vi "Dripline-agent.vi"() -> ()   [LabVIEW 2016]
panel:
  in  "message":string
  in  "target":string
  in  "timeout":dbl=10.0 format="%#_13g"
  in  "value":string
  in  "endpoint":string="broadcast.ping"
  in  "Request op":u16(ring)=1 items=["Set"=0, "Get"=1, "Send"=7, "Run"=8, "Command"=9]
  in  "Message type":u16(ring)=1 items=["alert", "request"]
  in  "host name":string="higgsino.physics.ucsb.edu"
  out "Array - String":string[](array[string])
  in  "error (in)":errorcluster
  out "error out":errorcluster
  # "alerts fields"
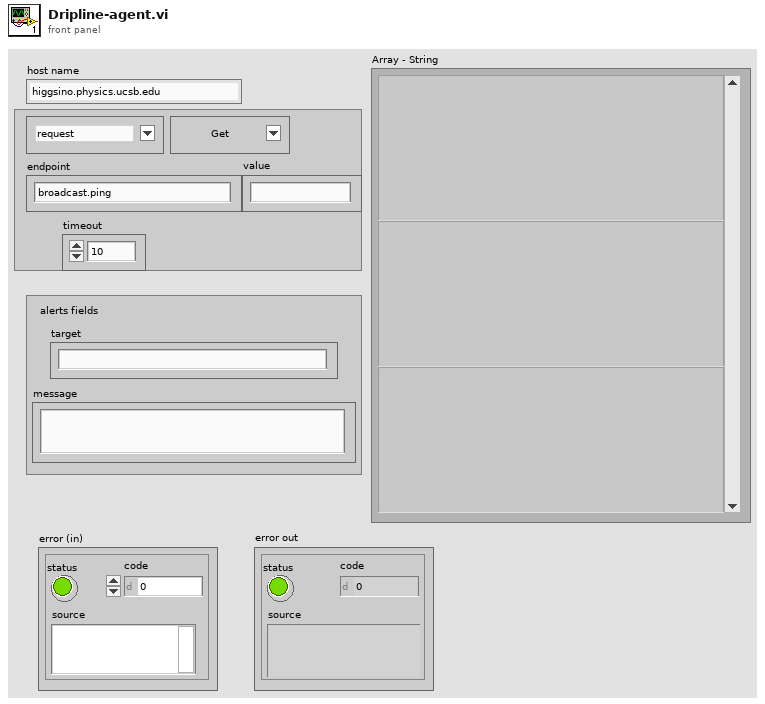
[diagram p1: front panel]
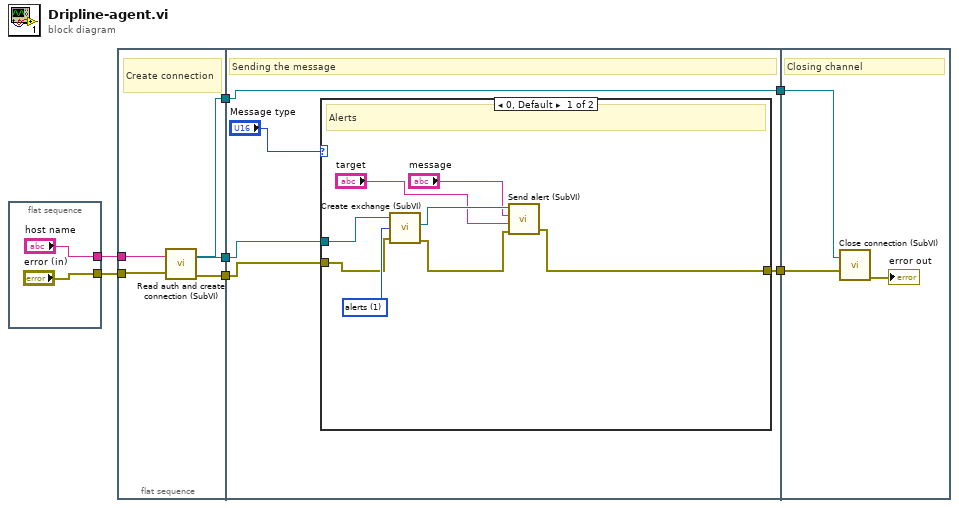
[diagram p0: block diagram]
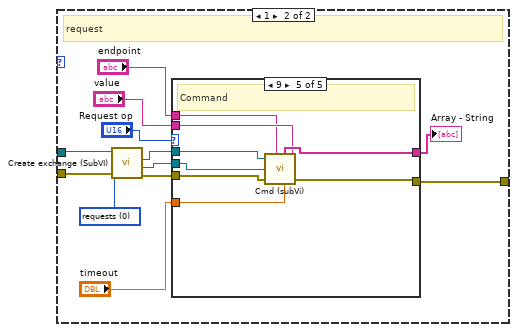
[diagram p2: hidden frame]
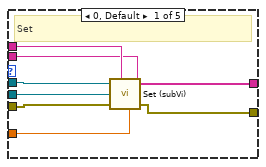
[diagram p3: hidden frame]
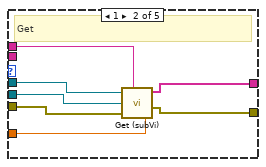
[diagram p4: hidden frame]
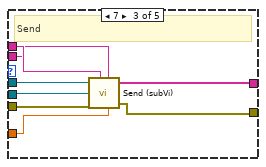
[diagram p5: hidden frame]
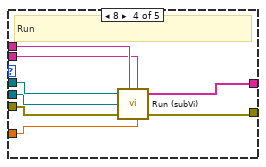
[diagram p6: hidden frame]
diagram:
  n1 = flat-sequence {
    tunnel: ["error (in)"] -> w5
    tunnel: ["host name"] -> w4
    frame #0 {
    }
  }
  n2 = flat-sequence {
    tunnel: [w10] -> w7
    tunnel: [w12] -> w6
    tunnel: w4 -> [w13]
    tunnel: w5 -> [w11]
    tunnel: [w10] -> w2
    tunnel: w6 -> [w18]
    tunnel: w7 -> [w15]
    tunnel: [w16] -> w3
    tunnel: w2 -> [w16]
    tunnel: [w14] -> w1
    tunnel: w3 -> [w79]
    tunnel: w1 -> [w78]
    frame #0 {
      # "Create connection"
      n3 = call "Read auth and create connection (SubVI).vi"("error in (no error)"=w11, "host name"=w13) -> ("error out"=w12:errorcluster, "Connection out"=w10:refnum<class "Connection.lvclass">)
    }
    frame #1 {
      # "Sending the message"
      n4 = case shown="0, Default" "Message type" {
        tunnel: w18 -> [w25 w31]
        tunnel: w15 -> [w23 w32]
        tunnel: [w19 w28] -> w14
        frame 0, Default {
          w26 = u16 1 items=["requests", "alerts"] ("exchange name")
          # "Alerts"
          n5 = call "Create exchange (SubVI).vi"("Connection in"=w23, "exchange name"=w26, "error in (no error)"=w25) -> ("Exchange.lvclass"=w24:refnum<class "Exchange.lvclass">, "error out"=w20:errorcluster)  [unwired: 2 out]
          n6 = call "Send alert (SubVI).vi"("error in (no error)"=w20, "target"="target", "message content"="message", "Exchange.lvclass"=w24) -> ("error out"=w19:errorcluster)  [unwired: 2 out]
        }
        frame 1 {
          w33 = u16 0 items=["requests", "alerts"] ("exchange name")
          # "request"
          n7 = call "Create exchange (SubVI).vi"("Connection in"=w32, "exchange name"=w33, "error in (no error)"=w31) -> ("Exchange.lvclass"=w38:refnum<class "Exchange.lvclass">, "Channel out"=w37:refnum<class "Channel.lvclass">, "error out"=w36:errorcluster)  [unwired: 1 out]
          n8 = case shown="9" "Request op" {
            tunnel: w38 -> [w43 w50 w61 w68 w73]
            tunnel: w37 -> [w42 w52 w60 w67 w72]
            tunnel: w36 -> [w41 w53 w59 w66 w71]
            tunnel: "endpoint" -> [w44 w51 w58 w64 w74]
            tunnel: "value" -> [w40 _ w55 w63 w75]
            tunnel: [w46 w49 w54 w62 w76] -> w29
            tunnel: [w45 w48 w56 w69 w77] -> w28
            tunnel: "timeout" -> [w39 w47 w57 w65 w70]
            frame 0, Default {
              # "Set"
              n9 = call "Set (subVi).vi"("Exchange.lvclass"=w43, "endpoint"=w44, "Channel in"=w42, "error in (no error)"=w41, "value"=w40, "timeout"=w39) -> ("Array - String"=w46:string[], "error out"=w45:errorcluster)  [unwired: 1 in, 1 out]
            }
            frame 1 {
              # "Get"
              n10 = call "Get (subVi).vi"("Exchange.lvclass"=w50, "endpoint"=w51, "Channel in"=w52, "error in (no error)"=w53, "timeout"=w47) -> ("Array - String"=w49:string[], "error IO"=w48:errorcluster)  [unwired: 1 in, 1 out]
            }
            frame 7 {
              # "Send"
              n11 = call "Send (subVi).vi"("Exchange.lvclass"=w61, "endpoint"=w58, "Channel in"=w60, "error in (no error)"=w59, "value"=w55, "timeout"=w57) -> ("Array - String"=w54:string[], "error IO"=w56:errorcluster)  [unwired: 1 in, 1 out]
            }
            frame 8 {
              # "Run"
              n12 = call "Run (subVi).vi"("Exchange.lvclass"=w68, "endpoint"=w64, "Channel in"=w67, "error in (no error)"=w66, "value"=w63, "timeout"=w65) -> ("Array - String"=w62:string[], "error IO"=w69:errorcluster)  [unwired: 1 in, 1 out]
            }
            frame 9 {
              # "Command"
              n13 = call "Cmd (subVi).vi"("Exchange.lvclass"=w73, "target"=w74, "Channel in"=w72, "error in (no error)"=w71, "value"=w75, "timeout"=w70) -> ("Array - String"=w76:string[], "error out"=w77:errorcluster)  [unwired: 1 in, 1 out]
            }
          }
          "Array - String" <- w29
        }
      }
    }
    frame #2 {
      # "Closing channel"
      n14 = call "Close connection (SubVI).vi"("error in (no error)"=w78, "Connection in"=w79) -> ("error out"=→"error out":errorcluster)  [unwired: 1 in]
    }
  }
